vi "Convert to Valid File Name.vi"(11 "File Name":string) -> (1 "Characters Removed?":bool, 3 "Valid File Name":string)   [LabVIEW 2020, in "MacroAssert.lvlib"]
doc: "Converts <B>File Name</B> to a valid file name by removing any characters that would not be allowed as per the Windows file naming conventions."
uses:
  MacroAssert.lvlib
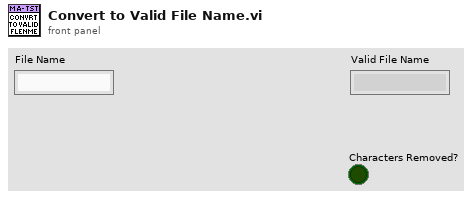
[diagram p1: front panel]
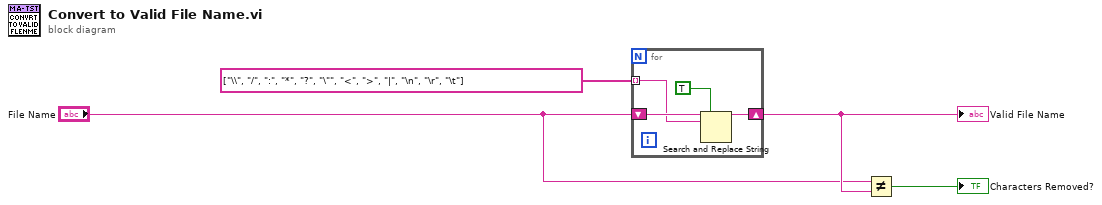
[diagram p0: block diagram]
diagram:
  n1 = for {
    tunnel: string[] ["\\", "/", ":", "*", "?", "\"", "<", ">", "|", "\n", "\r", "\t"] -> [w7] mode=indexing
    shift-right: [w6] -> w3
    shift-left: "File Name" -> [w8]
    n2 = Search and Replace String(replace all?=TRUE ("replace all? (F)"), input string=w8, search string=w7) -> (result string=w6:string)  [unwired: 5 in, 3 out]
  }
  "Valid File Name" <- w3
  n3 = Not Equal?(x="File Name", y=w3) -> (x != y?=→"Characters Removed?":bool)
